vi "Draw Arrow.vi"(6 "color":u32(colorbox)=12369084, 7 "picture info":T1={"picture size"={"Width"=500, "Height"=500}, "pixels per unit"=10.0}, 8 "global base position":cluster{"x":dbl, "y":dbl}, 9 "length":dbl, 10 "wheel frame angle (rad)":dbl, 11 "picture in":picture) -> (3 "picture out":picture)   [LabVIEW 2017, in "NI_Robotics_Steering Picture.lvlib"]
uses:
  <vilib>/robotics/Utilities/Visualization/Steering Visualization/Steering Picture/NI_Robotics_Steering Picture.lvlib
  <vilib>/robotics/Utilities/Visualization/Steering Visualization/Steering Picture/Picture Info.ctl
  <vilib>/Utility/miscctls.llb/LVBoundsTypeDef.ctl
  <vilib>/Analysis/coordinate.llb/2D Cartesian Coordinate Rotation (Array).vi
  <vilib>/Analysis/NI_AALPro.lvlib
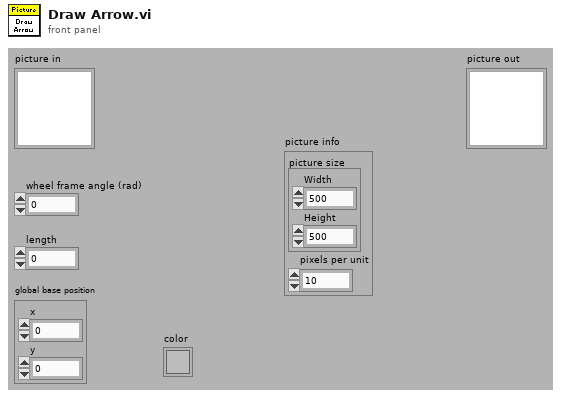
[diagram p1: front panel]
types:
  T1 = typedef "NI_Robotics_Steering Picture.lvlib/Picture Info.ctl" = cluster{"picture size":T2, "pixels per unit":dbl}
  T2 = typedef "LVBoundsTypeDef.ctl" = cluster{"Width":u32, "Height":u32}
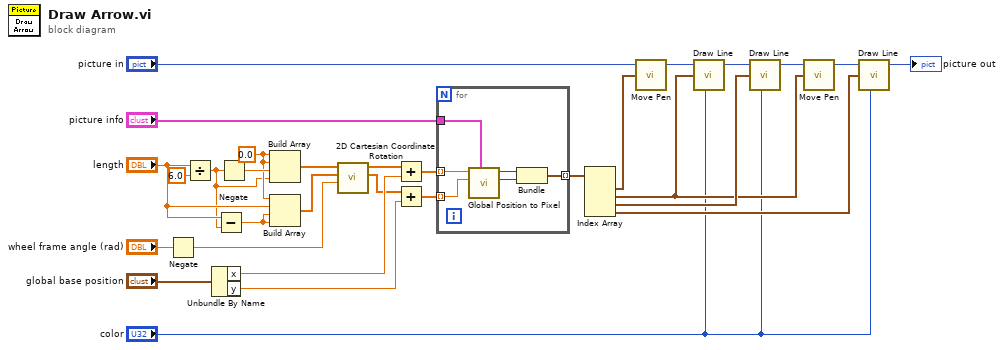
[diagram p0: block diagram]
diagram:
  w27 = 0.0 ("element")
  n1 = Negate(x="wheel frame angle (rad)") -> (-x=w21:dbl)
  n2 = Divide(x="length", y=6.0) -> (x/y=w25:dbl)
  n3 = Unbundle By Name("global base position") -> ("x"=w18:dbl, "y"=w16:dbl)
  n4 = Subtract(x="length", y=w25) -> (x-y=w24:dbl)
  n5 = Negate(x=w25) -> (-x=w28:dbl)
  n6 = Build Array(w27, w27, w28, w25) -> (w23:dbl[])
  n7 = Build Array(w27, "length", w24, w24) -> (w22:dbl[])
  n8 = call-poly <vilib>:"2D Cartesian Coordinate Rotation.vi"("theta"=w21, "Y"=w22, "X"=w23) -> ("Y Out"=w17:dbl[], "X Out"=w19:dbl[])  [unwired: 6 in, 1 out]
  n9 = Add(x=w19, y=w18) -> (x+y=w15:dbl[])
  n10 = Add(x=w17, y=w16) -> (x+y=w14:dbl[])
  n11 = for {
    tunnel: w15 -> [w36] mode=indexing
    tunnel: w14 -> [w35] mode=indexing
    tunnel: [w32] -> w13 mode=indexing
    tunnel: "picture info" -> [w31]
    n12 = call <vilib>:"Global Position to Pixel.vi"("picture info"=w31, "global y"=w35, "global x"=w36) -> ("pixel y"=w33:i16, "pixel x"=w34:i16)  [unwired: 7 in]
    n13 = Bundle("pixel x"=w34, "pixel y"=w33) -> (w32:cluster{"pixel x":i16, "pixel y":i16})  [unwired: 1 in]
  }
  n14 = Index Array(array=w13) -> (element #1=w12:cluster{"pixel x":i16, "pixel y":i16}, element #2=w6:cluster{"pixel x":i16, "pixel y":i16}, element #3=w8:cluster{"pixel x":i16, "pixel y":i16}, element #4=w4:cluster{"pixel x":i16, "pixel y":i16})  [unwired: 4 in]
  n15 = call <vilib>:"Move Pen.vi"("new position"=w12, "picture"="picture in") -> ("new picture"=w10:picture)  [unwired: 3 in]
  n16 = call <vilib>:"Draw Line.vi"("picture"=w10, "end point"=w6, "color(black)"="color") -> ("new picture"=w9:picture)  [unwired: 6 in]
  n17 = call <vilib>:"Draw Line.vi"("picture"=w9, "end point"=w8, "color(black)"="color") -> ("new picture"=w7:picture)  [unwired: 6 in]
  n18 = call <vilib>:"Move Pen.vi"("new position"=w6, "picture"=w7) -> ("new picture"=w5:picture)  [unwired: 3 in]
  n19 = call <vilib>:"Draw Line.vi"("picture"=w5, "end point"=w4, "color(black)"="color") -> ("new picture"=→"picture out":picture)  [unwired: 6 in]
